vi "Motor_tellposition.vi"(3 "error in (no error)":errorcluster, 4 "Conversion\n (steps/mm)":dbl[](array[numeric])=[12500.0, 31496.063, 31496.063, 31496.063] format="%#_13g", 5 "reference":refnum<k7>) -> (0 "error out":errorcluster, 1 "Position out":dbl[](array[numeric]), 2 "reference out":refnum<k7>)   [LabVIEW 2015]
uses:
  <vilib>/regexp/Match Regular Expression.xnode
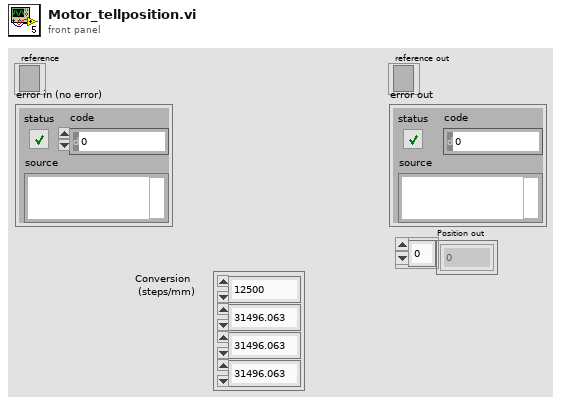
[diagram p1: front panel]
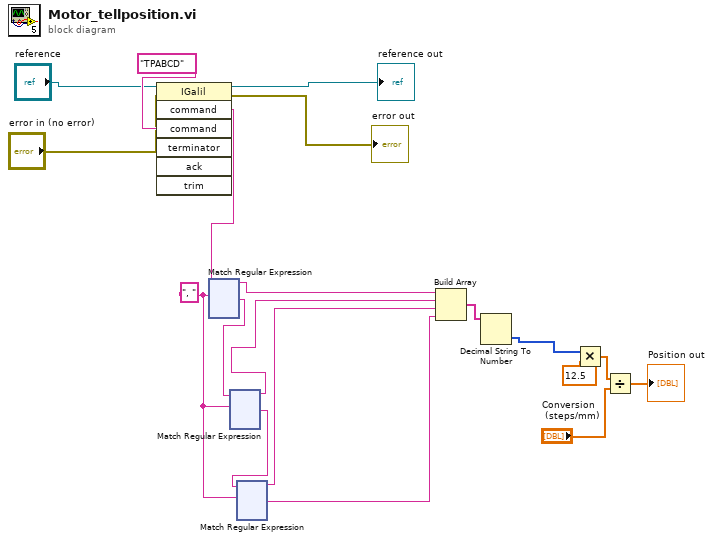
[diagram p0: block diagram]
diagram:
  w4 = ", " ("regular expression")
  n1 = invoke class="IGalil" method="command"(reference="reference", error in="error in (no error)", "command"="TPABCD") -> (reference out=→"reference out":refnum<k7>, error out=→"error out":errorcluster, "command"=w6:string)  [unwired: 4 in, 4 out]
  n2 = xnode "Match Regular Expression"("input string"=w6, "regular expression"=w4) -> ("before match"=w18:string, "after match"=w19:string)  [unwired: 4 in, 3 out]
  n3 = xnode "Match Regular Expression"("input string"=w19, "regular expression"=w4) -> ("before match"=w17:string, "after match"=w3:string)  [unwired: 4 in, 3 out]
  n4 = xnode "Match Regular Expression"("input string"=w3, "regular expression"=w4) -> ("before match"=w2:string, "after match"=w1:string)  [unwired: 4 in, 3 out]
  n5 = Build Array(w18, w17, w2, w1) -> (w16:string[])
  n6 = Decimal String To Number(string=w16) -> (number=w12:i32[])  [unwired: 2 in, 1 out]
  n7 = Multiply(x=w12, y=12.5) -> (x*y=w15:dbl[])
  n8 = Divide(x=w15, y="Conversion\n (steps/mm)") -> (x/y=→"Position out":dbl[])
